vi "CheckParameters.vi"(8 "error in (no error)":errorcluster, 10 "Parameters":dbl[](array[numeric]), 11 "EMTestCWS500N in":refnum<class "EMTestCWS500N.lvclass">) -> (0 "error out":errorcluster, 3 "EMTestCWS500N out":refnum<class "EMTestCWS500N.lvclass">)   [LabVIEW 2013, in "EMTestCWS500N.lvclass"]
uses:
  EMTestCWS500N.lvclass
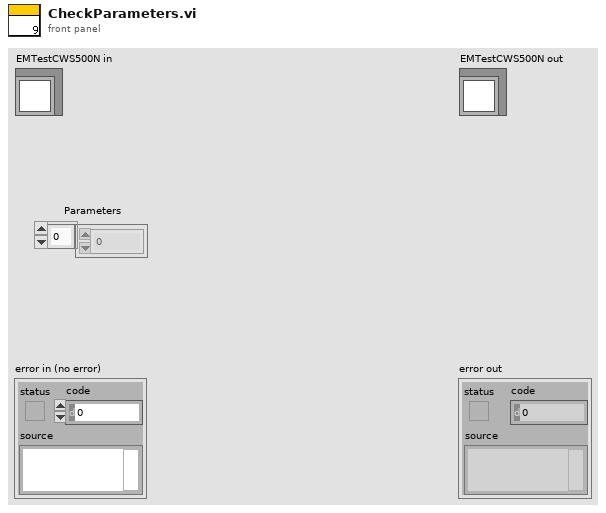
[diagram p1: front panel]
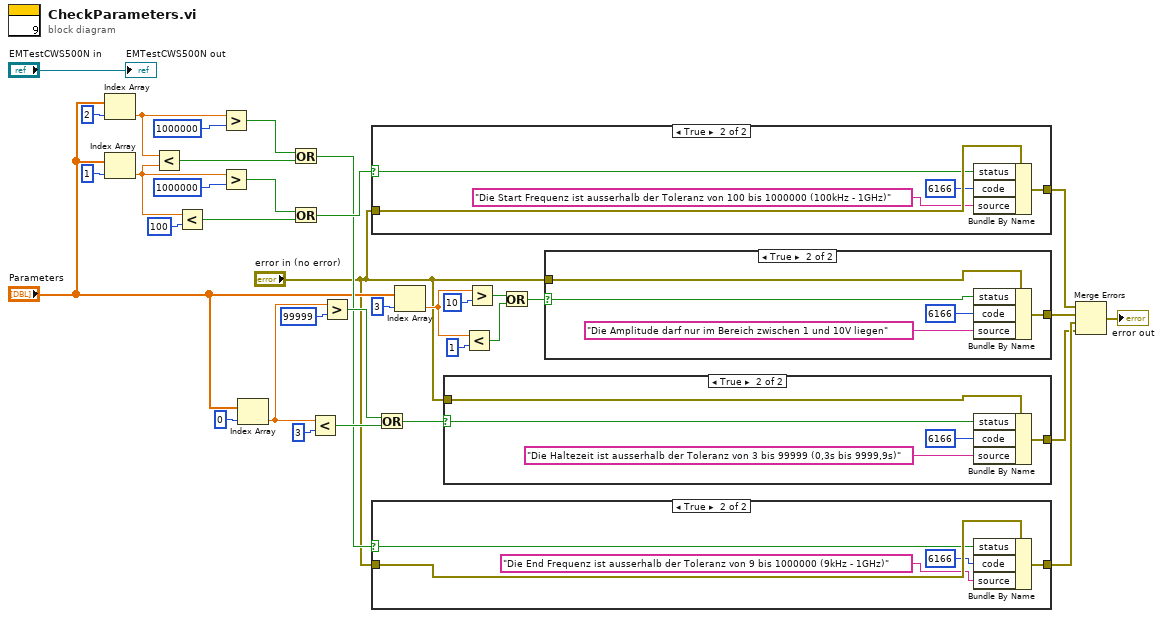
[diagram p0: block diagram]
diagram:
  n1 = Index Array(array="Parameters", index=2) -> (element=w34:dbl)
  n2 = Index Array(array="Parameters", index=1) -> (element=w1:dbl)
  n3 = Less?(x=w34, y=w1) -> (x < y?=w19:bool)
  n4 = Less?(x=w1, y=u32 100) -> (x < y?=w27:bool)
  n5 = Greater?(x=w34, y=u32 1000000) -> (0:w18:bool)
  n6 = Greater?(x=w1, y=u32 1000000) -> (0:w26:bool)
  n7 = Index Array(array="Parameters", index=0) -> (element=w35:dbl)
  n8 = Or(x=w18, y=w19) -> (x .or. y?=w10:bool)
  n9 = Or(x=w26, y=w27) -> (x .or. y?=w13:bool)
  n10 = Less?(x=w35, y=u32 3) -> (x < y?=w16:bool)
  n11 = Greater?(x=w35, y=u32 99999) -> (0:w15:bool)
  n12 = case shown="True" w13 {
    selector: w13 -> [_ w40]
    tunnel: "error in (no error)" -> [w36 w41]
    tunnel: [w36 w37] -> w9
    frame False {
    }
    frame True {
      n13 = Bundle By Name(cluster=w41, "status"=w40, "code"=6166, "source"="Die Start Frequenz ist ausserhalb der Toleranz von 100 bis 1000000 (100kHz - 1GHz)") -> (w37:errorcluster)
    }
  }
  n14 = case shown="True" w10 {
    selector: w10 -> [_ w46]
    tunnel: "error in (no error)" -> [w42 w47]
    tunnel: [w42 w43] -> w7
    frame False {
    }
    frame True {
      n15 = Bundle By Name(cluster=w47, "status"=w46, "code"=6166, "source"="Die End Frequenz ist ausserhalb der Toleranz von 9 bis 1000000 (9kHz - 1GHz)") -> (w43:errorcluster)
    }
  }
  n16 = Or(x=w15, y=w16) -> (x .or. y?=w11:bool)
  n17 = Index Array(array="Parameters", index=3) -> (element=w33:dbl)
  n18 = case shown="True" w11 {
    selector: w11 -> [_ w53]
    tunnel: [w48 w50] -> w6
    tunnel: "error in (no error)" -> [w48 w49]
    frame False {
    }
    frame True {
      n19 = Bundle By Name(cluster=w49, "status"=w53, "code"=6166, "source"="Die Haltezeit ist ausserhalb der Toleranz von 3 bis 99999 (0,3s bis 9999,9s)") -> (w50:errorcluster)
    }
  }
  n20 = Less?(x=w33, y=u32 1) -> (x < y?=w23:bool)
  n21 = Greater?(x=w33, y=u32 10) -> (0:w22:bool)
  n22 = Or(x=w22, y=w23) -> (x .or. y?=w12:bool)
  n23 = case shown="True" w12 {
    selector: w12 -> [_ w58]
    tunnel: "error in (no error)" -> [w54 w59]
    tunnel: [w54 w55] -> w8
    frame False {
    }
    frame True {
      n24 = Bundle By Name(cluster=w59, "status"=w58, "code"=6166, "source"="Die Amplitude darf nur im Bereich zwischen 1 und 10V liegen") -> (w55:errorcluster)
    }
  }
  n25 = Merge Errors(w9, w8, w7, w6) -> (→"error out":errorcluster)
  "EMTestCWS500N out" <- "EMTestCWS500N in"
